vi "FestoCPX.Valve(2out4in).vi"(4 "Delay [ms] (0)":u32, 6 "Timeout [ms] (5000)":u32=5000, 8 "error in (no error)":errorcluster, 9 "Position":T3, 10 "Valve outputs":T1[](array[typedef]), 11 "Inputs":T2[](array[typedef])) -> (0 "error out":errorcluster, 3 "Timeout?":bool)   [LabVIEW 2016]
uses:
  Station/Station.ValvePosition.ctl
  FestoCPX.DI.Signal.ctl
  FestoCPX.DO.Signal.ctl
panel:
  out "Aborted?":bool
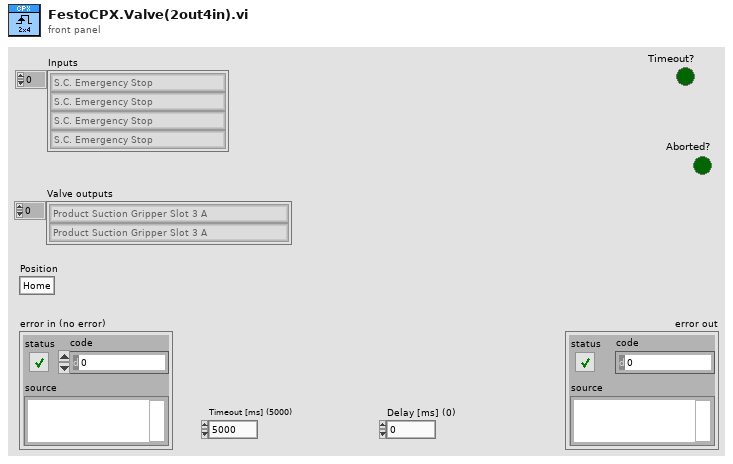
[diagram p1: front panel]
types:
  T1 = typedef "FestoCPX.DO.Signal.ctl" = enum16{"Safety Reset", "Air Main Valve", "Door Lock", "Button LED Start", "Button LED Stop", "Button LED Control", "Traffic LED Red", "Traffic LED Orange", "Traffic LED Green", "Horn", "Laser Interlock", "Laser Trigger", "Laser Fume Extractor", "Product Suction Gripper Slot 1 A", "Product Suction Gripper Slot 1 B", "Product Suction Gripper Slot 2 A", "Product Suction Gripper Slot 2 B", "Product Suction Gripper Slot 3 A", "Product Suction Gripper Slot 3 B", "Product Suction Gripper Slot 4 A", "Product Suction Gripper Slot 4 B", "Product Suction Gripper Final A", "Product Suction Gripper Final B", "Lamp", "Q1 Product Move Work", "Q1 Product Move Home", "Q2 Table Turn Work", "Q2 Table Turn Home", "Q3 Product Lift A", "Q3 Product Lift B", "Q4 Product Arm OK", "Q4 Product Arm NOK", "Q5 Product Arm Work", "Q6 Product BlowOut A", "Q6 Product BlowOut B"}
  T2 = typedef "FestoCPX.DI.Signal.ctl" = enum16{"S.C. Emergency Stop", "S.C. Side Door Close", "S.C. Front Door Close", "S.C. Front Door Secured", "Button Start", "Button Stop", "Button Control", "Product Move Home", "Product Move Work", "Table Position", "Table Lock", "Product Lift A Home", "Product Lift B Home", "Product Arm OK", "Product Arm NOK", "Product Arm Work", "Revolver ID 1", "Revolver ID 2", "Revolver ID 3", "Revolver ID 4", "Revolver ID 5", "Air Pressure Inside", "Air Pressure Inlet", "Product Slot 1 A Present", "Product Slot 1 B Present", "Product Slot 2 A Present", "Product Slot 2 B Present", "Product Slot 3 A Present", "Product Slot 3 B Present", "Product Slot 4 A Present", "Product Slot 4 B Present", "Product Final A Present", "Product Final B Present", "Product Output A Present", "Product Output B Present", "Product Container OK Present", "Product Container NOK Present", "Fork ID 1", "Fork ID 2"}
  T3 = typedef "Station.ValvePosition.ctl" = enum16{"Home", "Work"}
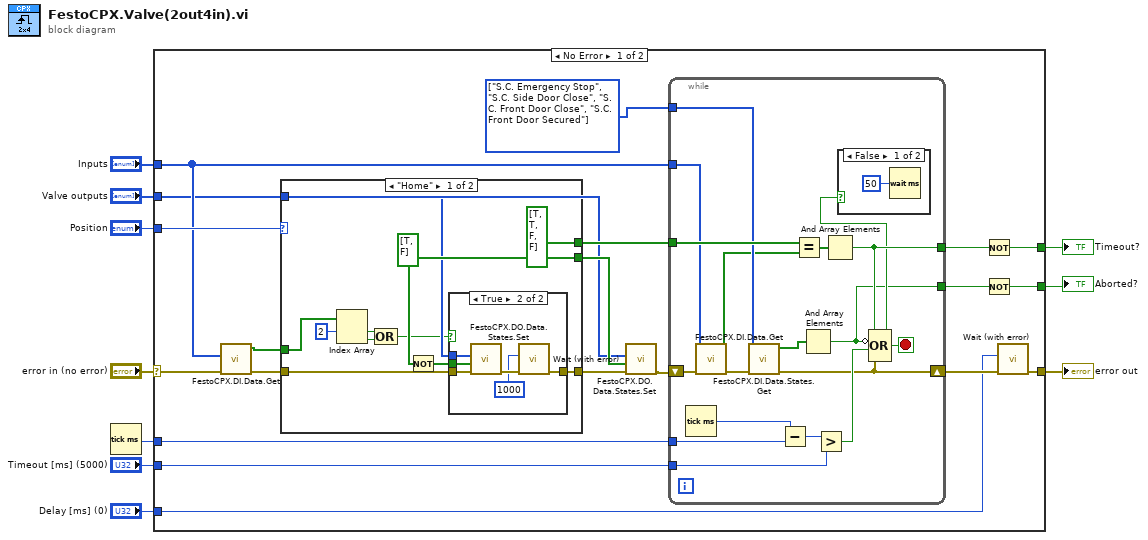
[diagram p0: block diagram]
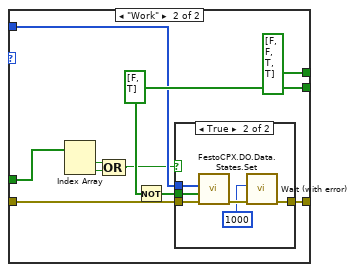
[diagram p4: hidden frame]
diagram:
  n1 = Tick Count (ms)() -> (millisecond timer value=w6:u32)
  n2 = case shown="No Error" "error in (no error)" {
    selector: "error in (no error)" -> [w18 w84]
    tunnel: "Position" -> [w23 _]
    tunnel: [w25 w84] -> w9
    tunnel: [w28 _] -> w8
    tunnel: w6 -> [w30 _]
    tunnel: "Timeout [ms] (5000)" -> [w29 _]
    tunnel: "Inputs" -> [w16 _]
    tunnel: "Valve outputs" -> [w15 _]
    tunnel: "Delay [ms] (0)" -> [w24 _]
    tunnel: [w12 _] -> w1
    frame No Error {
      w14 = T2[] [enum."S.C. Emergency Stop", enum."S.C. Side Door Close", enum."S.C. Front Door Close", enum."S.C. Front Door Secured"] items=["S.C. Emergency Stop", "S.C. Side Door Close", "S.C. Front Door Close", "S.C. Front Door Secured", "Button Start", "Button Stop", "Button Control", "Product Move Home", "Product Move Work", "Table Position", "Table Lock", "Product Lift A Home", "Product Lift B Home", "Product Arm OK", "Product Arm NOK", "Product Arm Work", "Revolver ID 1", "Revolver ID 2", "Revolver ID 3", "Revolver ID 4", "Revolver ID 5", "Air Pressure Inside", "Air Pressure Inlet", "Product Slot 1 A Present", "Product Slot 1 B Present", "Product Slot 2 A Present", "Product Slot 2 B Present", "Product Slot 3 A Present", "Product Slot 3 B Present", "Product Slot 4 A Present", "Product Slot 4 B Present", "Product Final A Present", "Product Final B Present", "Product Output A Present", "Product Output B Present", "Product Container OK Present", "Product Container NOK Present", "Fork ID 1", "Fork ID 2"] ("CPX.DI")
      n3 = call-poly "FestoCPX.DI.Data.Get.vi"("error in (no error)"=w18, "CPX.DI"=w16) -> ("error out"=w17:errorcluster, "State"=w11:bool[])  [unwired: 5 in, 3 out]
      n4 = case shown="\"Home\"" w23 {
        tunnel: [bool[] [TRUE, TRUE, FALSE, FALSE] bool[] [FALSE, FALSE, TRUE, TRUE]] -> w22
        tunnel: w17 -> [w59 w76]
        tunnel: [w58 w75] -> w21
        tunnel: [w55 w72] -> w19
        tunnel: w15 -> [w54 w71]
        tunnel: w11 -> [w51 w67]
        frame "Home" {
          w55 = bool[] [TRUE, FALSE]
          n5 = Index Array(array=w51, index #1=2 ("index")) -> (element #1=w53:bool, element #2=w52:bool)  [unwired: 1 in]
          n6 = Compound Arithmetic op=OR(w53, w52) -> (w50:bool)
          n7 = Not(x=w55) -> (.not. x?=w56:bool[])
          n8 = case shown="True" w50 {
            tunnel: w59 -> [w60 w62]
            tunnel: [w60 w61] -> w58
            tunnel: w56 -> [_ w64]
            tunnel: w54 -> [_ w63]
            frame False {
            }
            frame True {
              n9 = call "FestoCPX.DO.Data.States.Set.vi"("error in (no error)"=w62, "State"=w64, "CPX.DO"=w63) -> ("error out"=w66:errorcluster)  [unwired: 8 in]
              n10 = call "Wait (with error).vi"("error in (no error)"=w66, "milliseconds to wait"=u32 1000 ("Delay [ms] (0)")) -> ("error out"=w61:errorcluster)  [unwired: 8 in, 1 out]
            }
          }
        }
        frame "Work" {
          w72 = bool[] [FALSE, TRUE]
          n11 = Index Array(array=w67) -> (element #1=w70:bool, element #2=w69:bool)  [unwired: 2 in]
          n12 = Compound Arithmetic op=OR(w70, w69) -> (w68:bool)
          n13 = Not(x=w72) -> (.not. x?=w73:bool[])
          n14 = case shown="True" w68 {
            tunnel: w76 -> [w77 w80]
            tunnel: [w77 w81] -> w75
            tunnel: w73 -> [_ w79]
            tunnel: w71 -> [_ w78]
            frame False {
            }
            frame True {
              n15 = call "FestoCPX.DO.Data.States.Set.vi"("error in (no error)"=w80, "State"=w79, "CPX.DO"=w78) -> ("error out"=w83:errorcluster)  [unwired: 8 in]
              n16 = call "Wait (with error).vi"("error in (no error)"=w83, "milliseconds to wait"=u32 1000 ("Delay [ms] (0)")) -> ("error out"=w81:errorcluster)  [unwired: 8 in, 1 out]
            }
          }
        }
      }
      n17 = call "FestoCPX.DO.Data.States.Set.vi"("error in (no error)"=w21, "State"=w19, "CPX.DO"=w15) -> ("error out"=w20:errorcluster)  [unwired: 8 in]
      n18 = while {
        shift-right: [w36] -> w26
        shift-left: w20 -> [w47]
        tunnel: w16 -> [w35]
        tunnel: [w39] -> w27
        tunnel: w30 -> [w45]
        tunnel: w29 -> [w43]
        tunnel: w22 -> [w42]
        tunnel: w14 -> [w34]
        tunnel: [w33] -> w13
        stop <- w38 stop-if-true
        n19 = Tick Count (ms)() -> (millisecond timer value=w46:u32)
        n20 = call-poly "FestoCPX.DI.Data.Get.vi"("error in (no error)"=w47, "CPX.DI"=w35) -> ("error out"=w37:errorcluster, "State"=w32:bool[])  [unwired: 5 in, 3 out]
        n21 = call "FestoCPX.DI.Data.States.Get.vi"("error in (no error)"=w37, "CPX.DI"=w34) -> ("error out"=w36:errorcluster, "State"=w31:bool[])  [unwired: 5 in, 3 out]
        n22 = Subtract(x=w46, y=w45) -> (x-y=w44:u32)
        n23 = Equal?(x=w42, y=w32) -> (x = y?=w41:bool[])
        n24 = And Array Elements(Boolean array=w31) -> (logical AND=w33:bool)
        n25 = Greater?(x=w44, y=w43) -> (0:w40:bool)
        n26 = And Array Elements(Boolean array=w41) -> (logical AND=w39:bool)
        n27 = Compound Arithmetic op=OR(w39, invert w33, w40, w36) -> (w38:bool)
        n28 = case shown="False" w38 {
          frame False {
            n29 = Wait (ms)(milliseconds to wait=u32 50) -> ()  [unwired: 1 out]
          }
          frame True {
          }
        }
      }
      n30 = Not(x=w27) -> (.not. x?=w28:bool)
      n31 = Not(x=w13) -> (.not. x?=w12:bool)
      n32 = call "Wait (with error).vi"("error in (no error)"=w26, "milliseconds to wait"=w24) -> ("error out"=w25:errorcluster)  [unwired: 8 in, 1 out]
    }
    frame Error {
    }
  }
  "error out" <- w9
  "Timeout?" <- w8
  "Aborted?" <- w1
